vi "TestTPullse.vi"() -> ()   [LabVIEW 2022 SP3, in "BinarySignalProcessClass.lvclass"]
uses:
  BinarySignalProcessClass.lvclass
  BinarySignalProcessClass.lvclass/BinarySignalProcessClass.ctl
panel:
  out "Waveform Chart":u8(graph)
  in  "stop":bool
  in  "input":bool
  in  "TPulse":i32
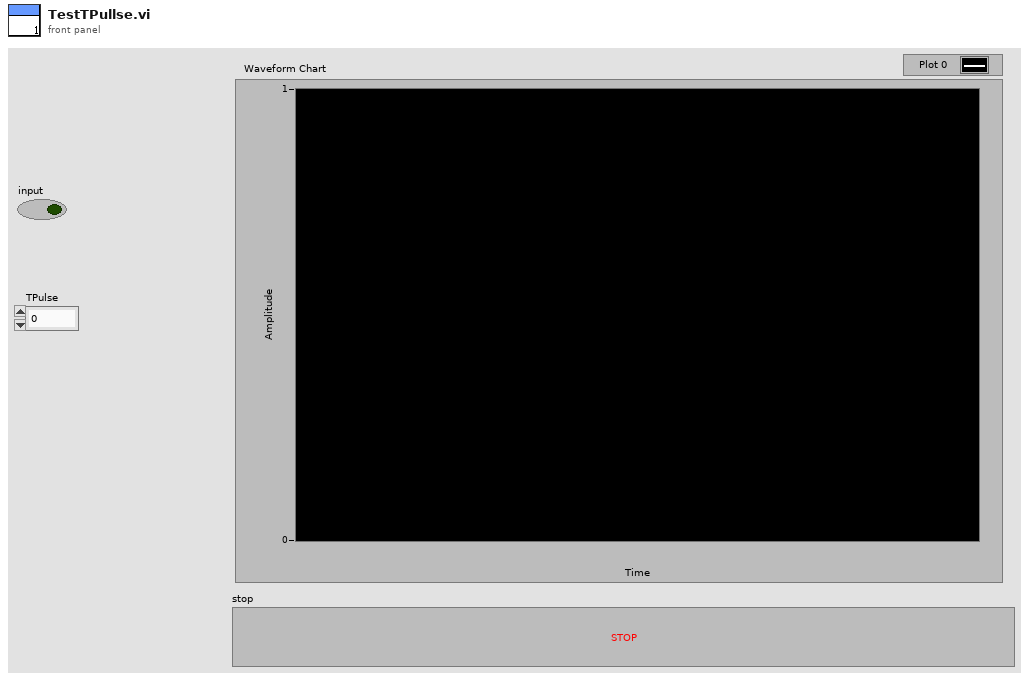
[diagram p1: front panel]
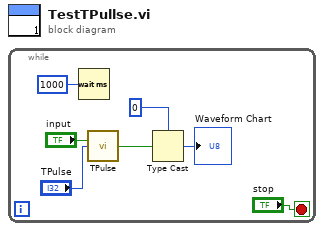
[diagram p0: block diagram]
diagram:
  n1 = while {
    stop <- "stop" stop-if-true
    n2 = Wait (ms)(milliseconds to wait=u32 1000) -> ()  [unwired: 1 out]
    n3 = call "TPulse.vi"("input"="input", "TPulse"="TPulse") -> ("output"=w2:bool)  [unwired: 12 in, 1 out]
    n4 = Type Cast(type=u8 0, x=w2) -> (*(type *) &x=→"Waveform Chart":u8)
  }
